vi "port_write.vi"(8 "error in (no error)":errorcluster, 10 "write buffer":string, 11 "VISA Refnum in":refnum<visa-resource-name>) -> (0 "error out":errorcluster, 3 "VISA Refnum out":refnum<visa-resource-name>)   [LabVIEW 2024]
uses:
  <vilib>/Utility/error.llb/Trim Whitespace One-Sided.vi
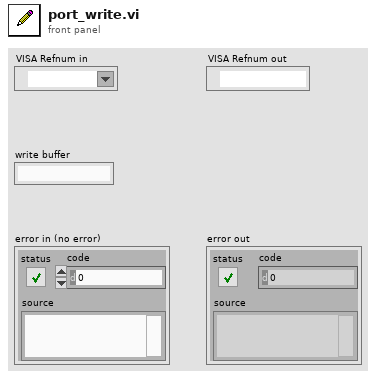
[diagram p1: front panel]
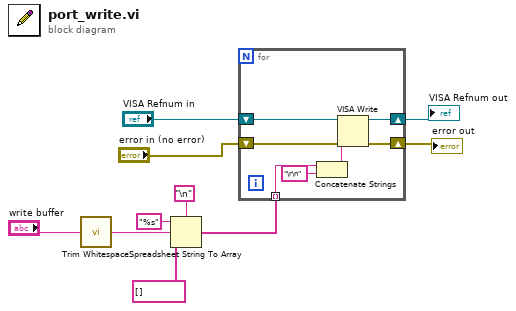
[diagram p0: block diagram]
diagram:
  n1 = call <vilib>:"Trim Whitespace.vi"("string"="write buffer") -> ("trimmed string"=w6:string)  [unwired: 1 in]
  n2 = Spreadsheet String To Array(delimiter (Tab)="\n" ("search string"), format string="%s", spreadsheet string=w6, array type (2D Dbl)=string[] []) -> (array=w7:string[])
  n3 = for {
    shift-right: [w11] -> w2
    shift-left: "error in (no error)" -> [w13]
    shift-right: [w12] -> w3
    shift-left: "VISA Refnum in" -> [w15]
    tunnel: w7 -> [w16] mode=indexing
    n4 = Concatenate Strings(w16, "\r\n" ("string")) -> (w14:string)
    n5 = VISA Write(VISA resource name=w15, write buffer=w14, error in (no error)=w13) -> (VISA resource name out=w12:refnum<visa-resource-name>, error out=w11:errorcluster)  [unwired: 1 out]
  }
  "error out" <- w2
  "VISA Refnum out" <- w3
